vi "Save Setting.vi"(8 "error in":errorcluster, 10 "Element Labels":string[](array[string]), 11 "Class in":refnum<class>) -> (0 "error out":errorcluster, 3 "Class out":refnum<class>)   [LabVIEW 2023, in "Label-Driven UI.lvlib"]
doc: "어플리케이션 디렉토리/Config에 입력한 라벨(들)에 해당하는 컨트롤(들)이 가진 값을 저장합니다."
uses:
  Label-Driven UI.lvlib
  3c837dc7-2e1d-4e05-acbb-346ed34a3f0b.vi
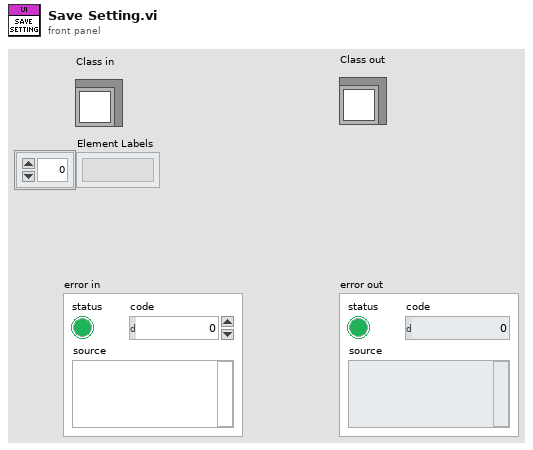
[diagram p1: front panel]
types:
  T1 = enum16{"big-endian, network order", "native, host order", "little-endian"}
  T2 = enum16{"open", "replace", "create", "open or create", "replace or create", "replace or create with confirmation"}
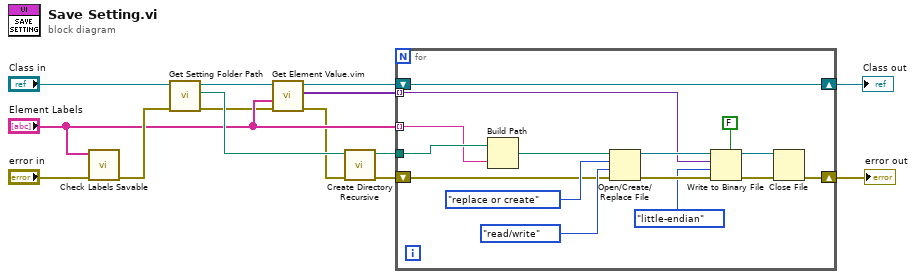
[diagram p0: block diagram]
diagram:
  n1 = call "Check Labels Savable.vi"("error in"="error in", "Element Labels"="Element Labels") -> ("error out"=w7:errorcluster)  [unwired: 9 in]
  n2 = call "Get Setting Folder Path.vi"("error in (no error)"=w7, "LabVIEW Object in"="Class in") -> ("error out"=w2:errorcluster, "appended path"=w9:path, "LabVIEW Object out"=w6:refnum<class>)  [unwired: 7 in]
  n3 = call "Get Element Value.vim"("error in"=w2, "Label"="Element Labels", "Class in"=w6) -> ("error out"=w1:errorcluster, "Value"=w4:variant[], "Class out"=w5:refnum<class>)  [unwired: 6 in]
  n4 = call <vilib>:"Create Directory Recursive.vi"("error in (no error)"=w1, "directory"=w9) -> ("error out"=w12:errorcluster, "directory copy"=w13:path)  [unwired: 3 in, 1 out]
  n5 = for {
    shift-right: [w17] -> w11
    shift-left: w5 -> [w17]
    tunnel: w13 -> [w21]
    tunnel: "Element Labels" -> [w19] mode=indexing
    shift-right: [w18] -> w10
    shift-left: w12 -> [w16]
    tunnel: w4 -> [w15] mode=indexing
    n6 = Build Path(base path=w21, name or relative path=w19) -> (appended path=w20:path)
    n7 = Open/Create/Replace File(file path (use dialog)=w20, error in=w16, operation (0:open)=T2."replace or create", access (0:read/write)=enum16{"read/write", "read-only", "write-only"}."read/write") -> (refnum out=w24:refnum<file>, error out=w27:errorcluster)  [unwired: 2 in, 1 out]
    n8 = Write to Binary File(file (use dialog)=w24, data=w15, error in=w27, 5:FALSE ("prepend array or string size? (T)"), 9:T1."little-endian" ("byte order (0:big-endian, network order)")) -> (refnum out=w22:refnum<file>, error out=w23:errorcluster)  [unwired: 1 in, 1 out]
    n9 = Close File(refnum=w22, error in=w23) -> (error out=w18:errorcluster)  [unwired: 1 out]
  }
  "Class out" <- w11
  "error out" <- w10
